vi "Calculate Number of Text Rows.vi"(0 "Library Path":path, 5 "Number of Pixel Rows in Icon":i32, 7 "Icon Height":i32=30) -> (4 "Number of Text Rows":i32, 6 "Blank Line 1 Text":bool)   [LabVIEW 2024, in "Text-Based VI Icon.lvlib"]
uses:
  <vilib>/LabVIEW Icon API/Set Text Icon/Text-Based VI Icon.lvlib
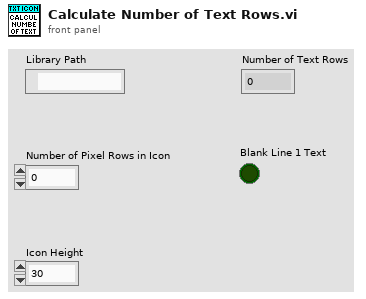
[diagram p1: front panel]
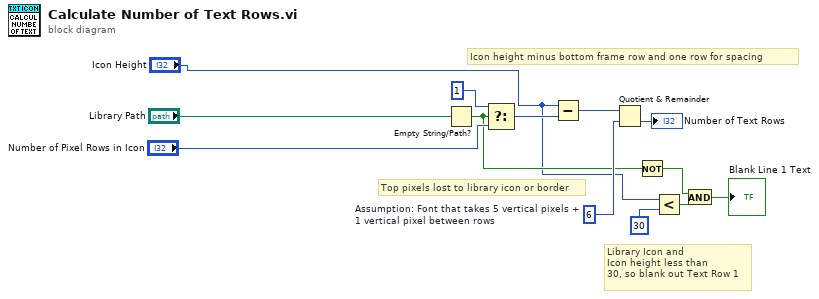
[diagram p0: block diagram]
diagram:
  w13 = 6  # Assumption: Font that takes 5 vertical pixels + 1 vertical pixel between rows
  # "Library Icon and\nIcon height less than\n30, so blank out Text Row 1"
  # "Icon height minus bottom frame row and one row for spacing"
  # "Top pixels lost to library icon or border"
  n1 = Empty String/Path?(string/path="Library Path") -> (empty?=w2:bool)
  n2 = Select(t=1, s=w2, f="Number of Pixel Rows in Icon") -> (s? t:f=w8:i32)
  n3 = Subtract(x="Icon Height", y=w8) -> (x-y=w7:i32)
  n4 = Quotient & Remainder(x=w7, y=w13) -> (floor(x/y)=→"Number of Text Rows":i32)  [unwired: 1 out]
  n5 = Not(x=w2) -> (.not. x?=w3:bool)
  n6 = Less?(x="Icon Height", y=30) -> (x < y?=w5:bool)
  n7 = And(x=w3, y=w5) -> (x .and. y?=→"Blank Line 1 Text":bool)
